vi "ClientTest.vi"() -> ()   [LabVIEW 2019]
panel:
  in  "port":u16
  in  "remote IP":string
  out "RawData":string
  in  "End":string="</CurrentMeasure>"
  out "CurrentData":string
  in  "Start":string="<CurrentMeasure>"
  out "error out TCPIP":errorcluster
  out "TM State Machine":string
  out "TM State Machine update time":timestamp
  out "TMisConnected":bool
  out "stopped":bool
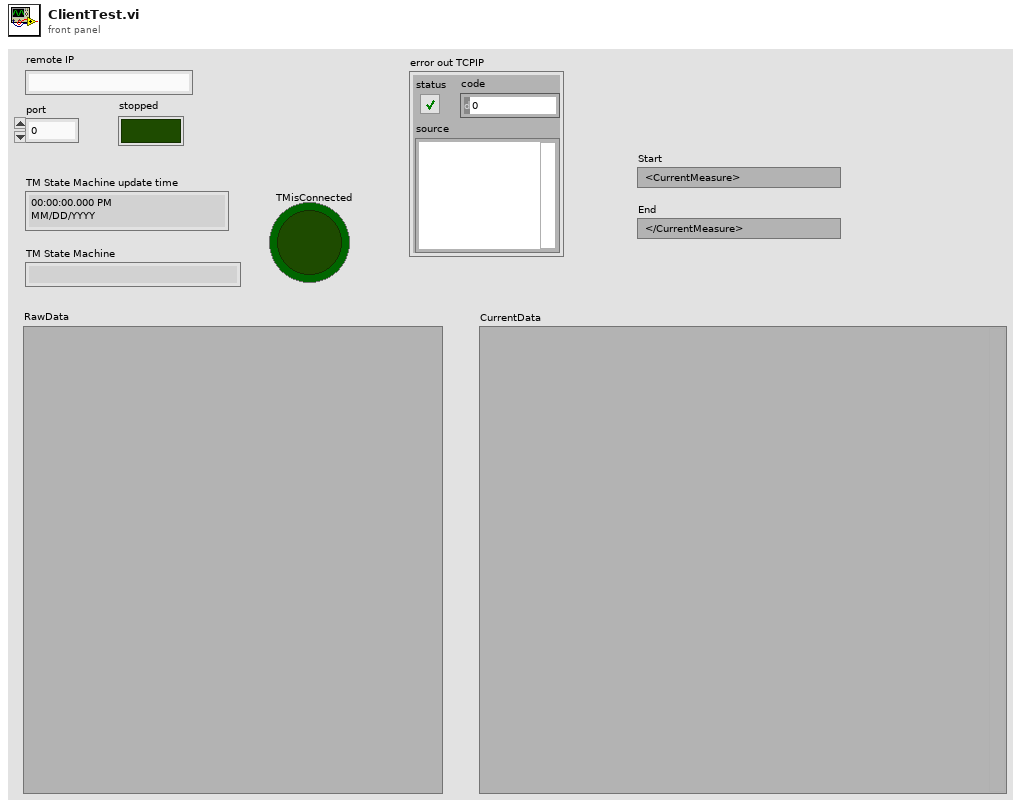
[diagram p1: front panel]
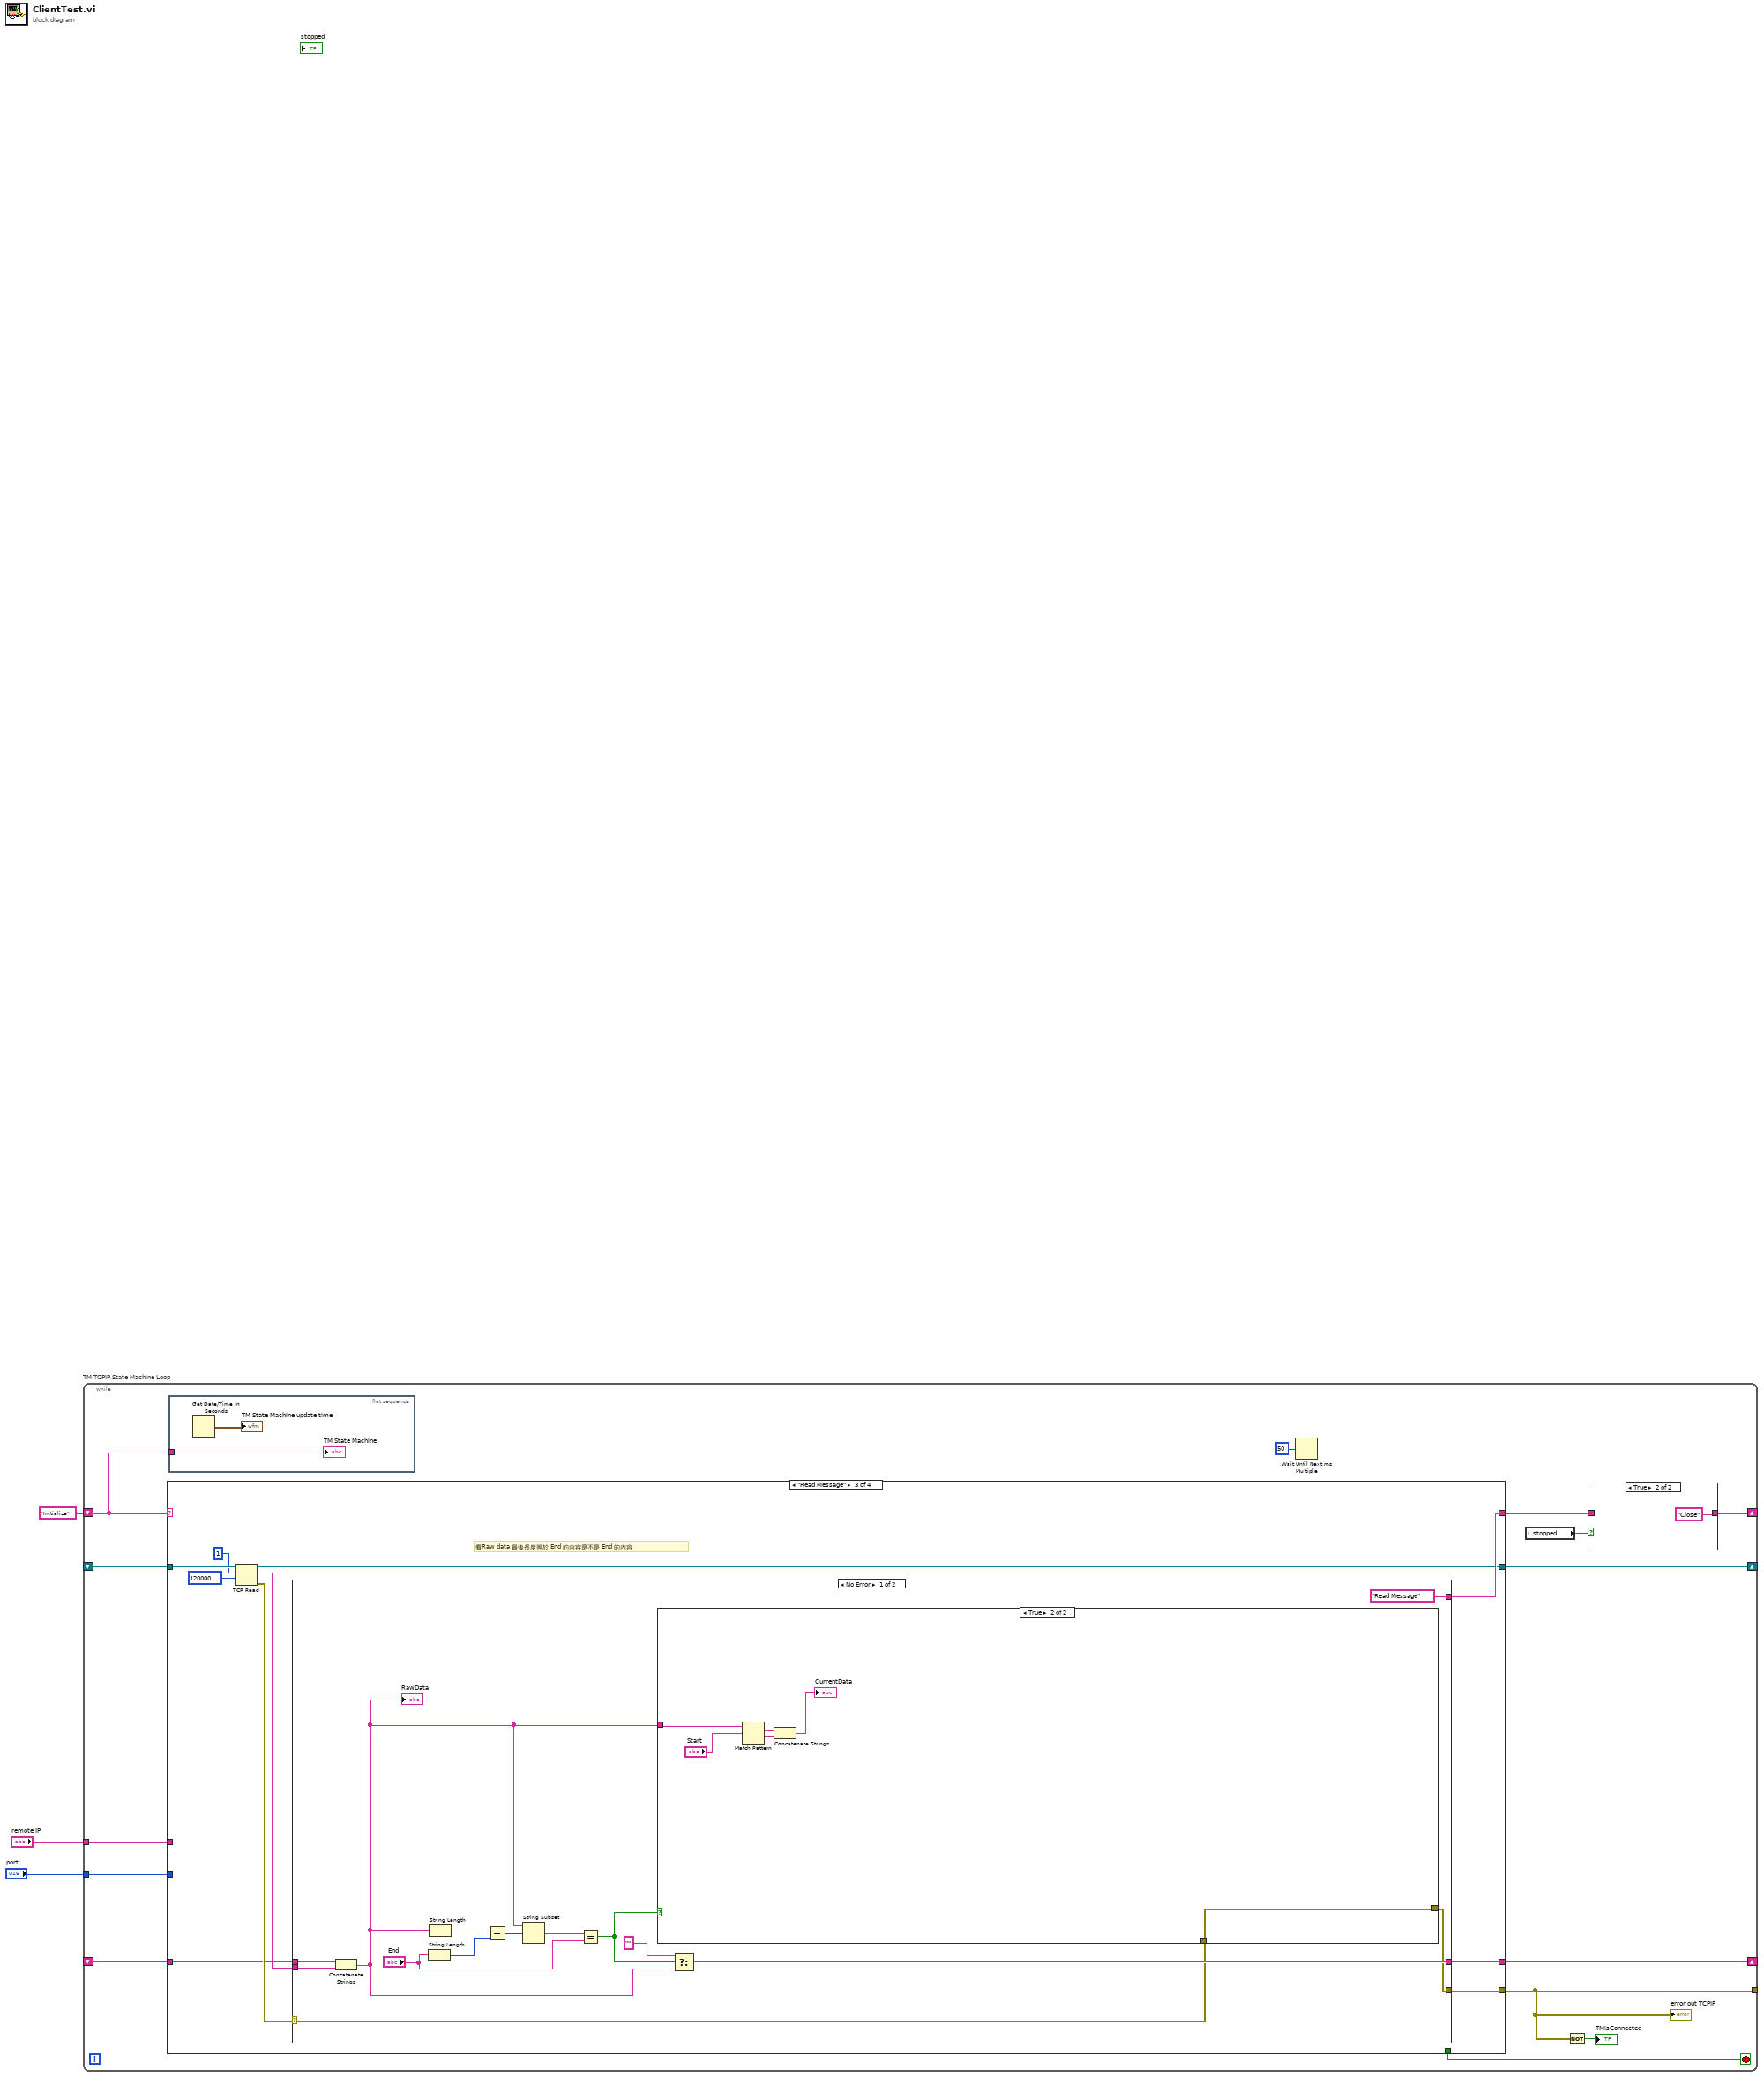
[diagram p0: block diagram]
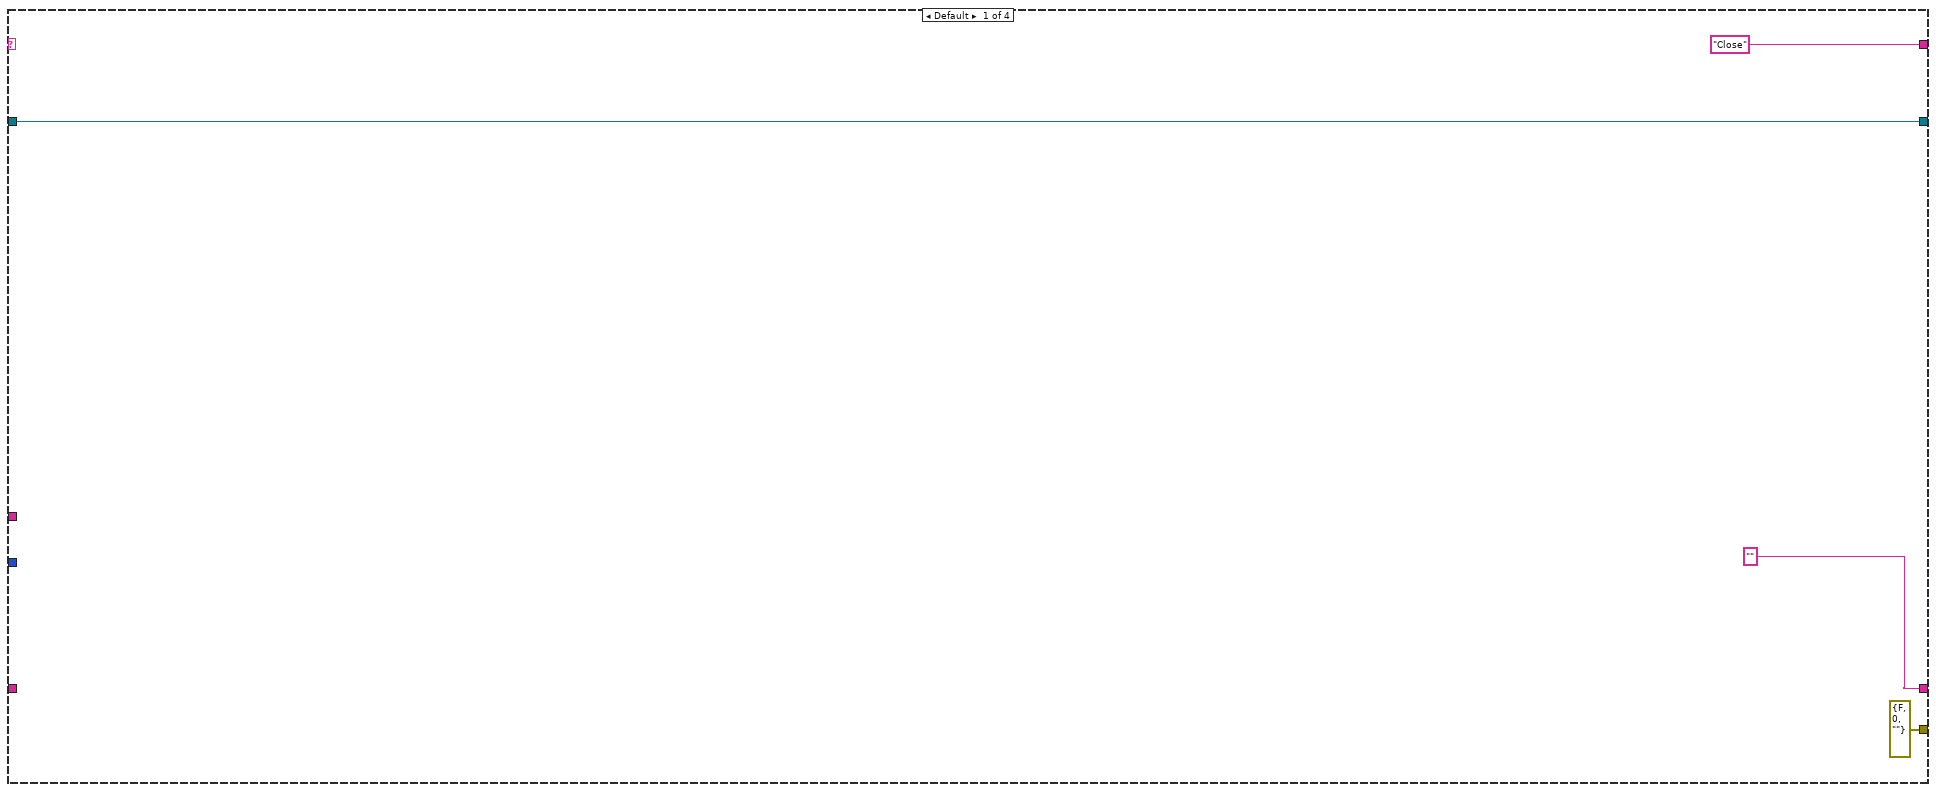
[diagram p3: hidden frame]
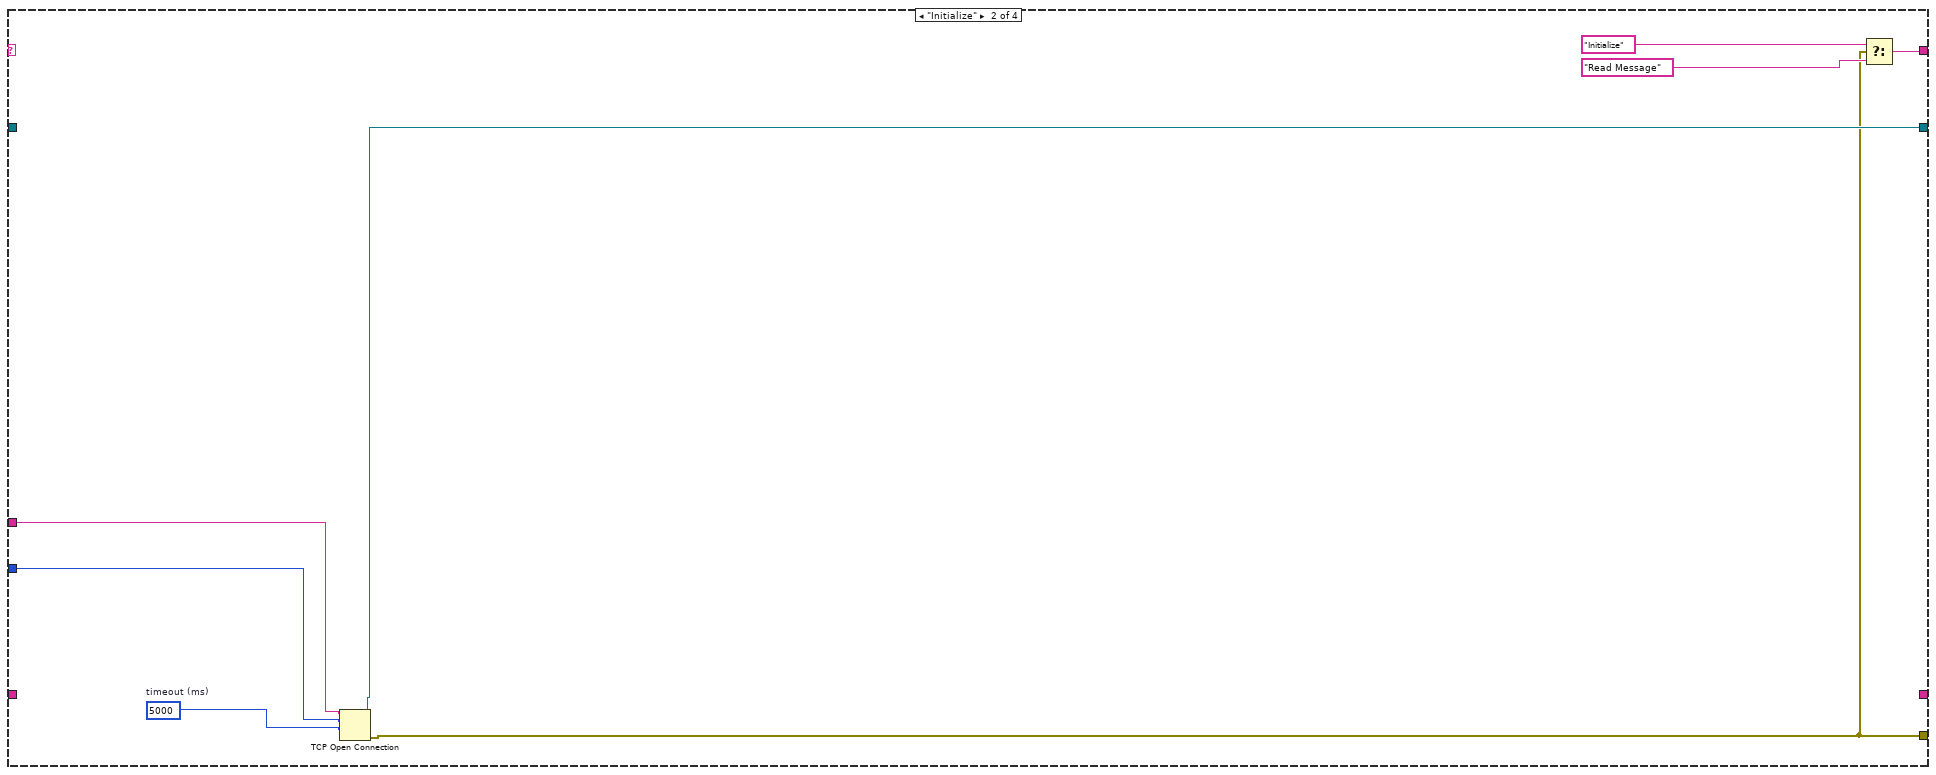
[diagram p4: hidden frame]
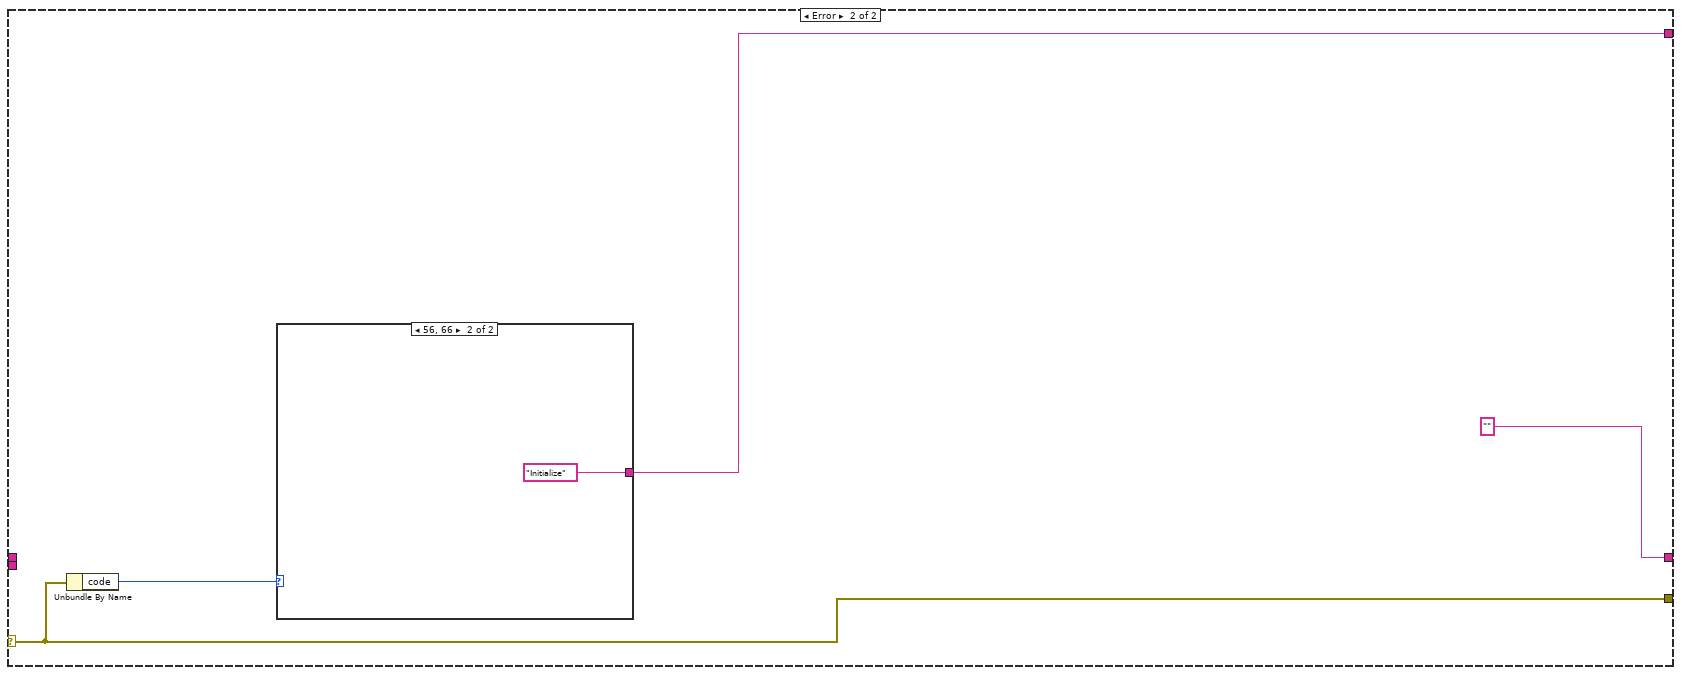
[diagram p6: hidden frame]
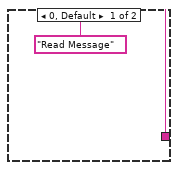
[diagram p7: hidden frame]
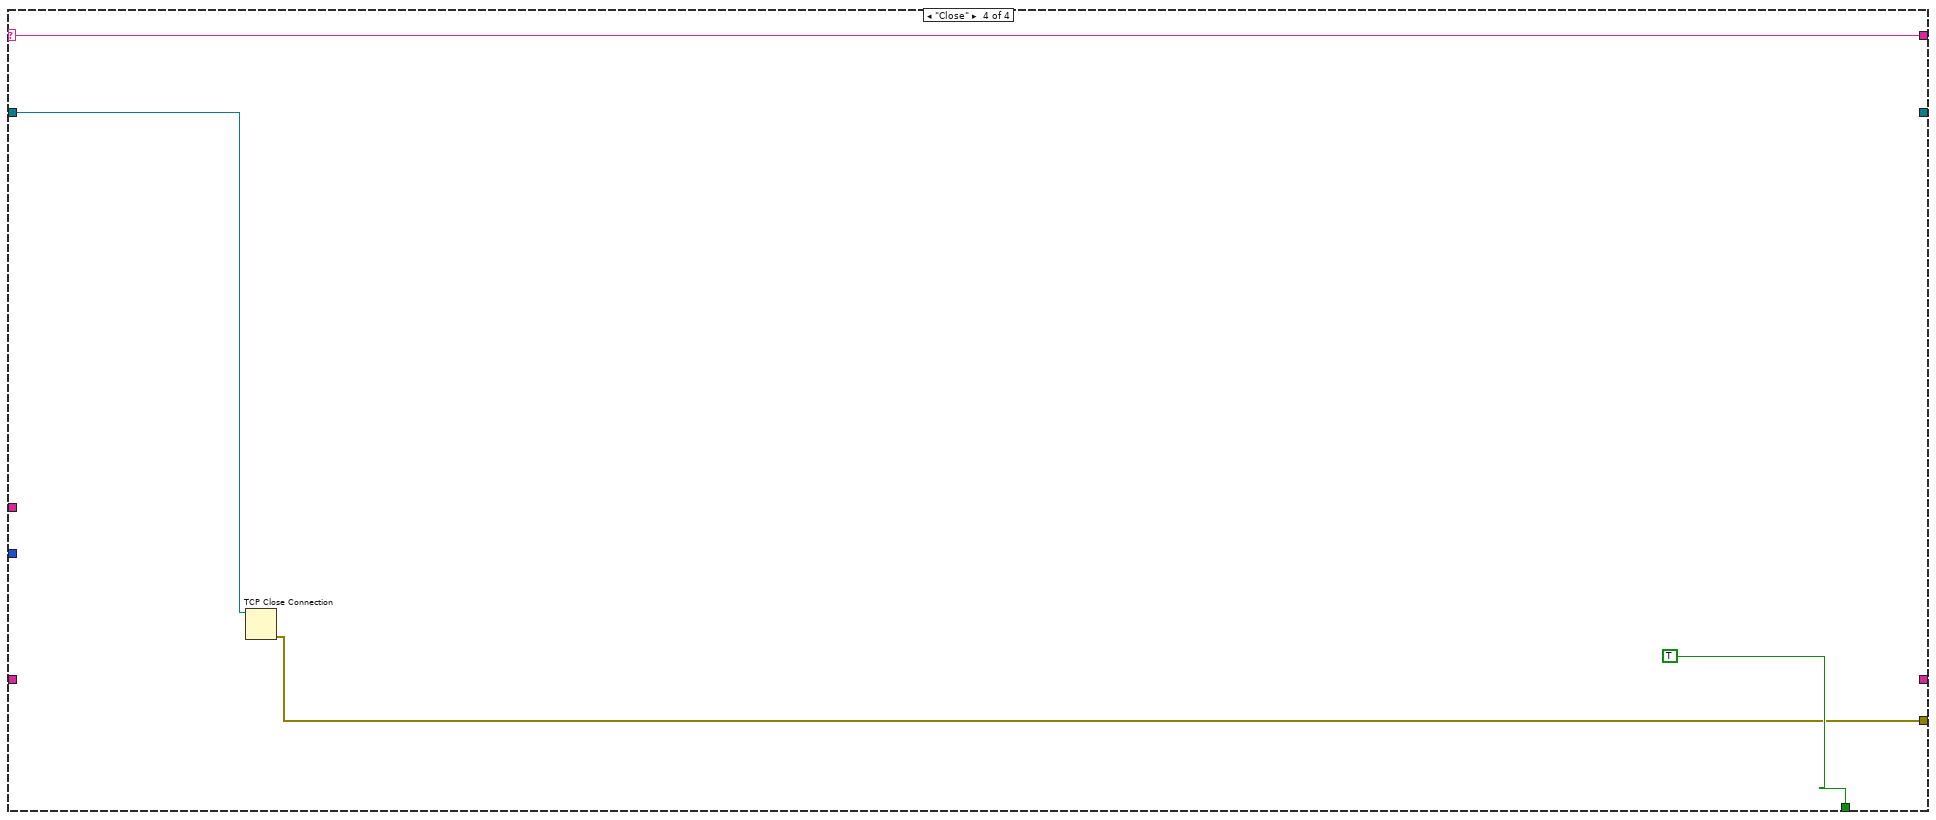
[diagram p8: hidden frame]
diagram:
  n1 = while "TM TCPIP State Machine Loop" {
    shift-right: [w10] -> _
    shift-left: "Initialize" -> [w9]
    tunnel: [w8] -> _
    shift-right: [w17] -> _
    shift-left: _ -> [w16]
    shift-right: [w15] -> _
    shift-left: _ -> [w14]
    tunnel: "remote IP" -> [w7]
    tunnel: "port" -> [w6]
    stop <- w13 stop-if-true
    n2 = case shown="\"Read Message\"" w9 {
      selector: w9 -> [_ _ _ w72]
      tunnel: ["Close" w31 w39 w72] -> w11
      tunnel: [errorcluster {"status"=FALSE, "code"=0, "source"=""} ("error out") w26 w34 w71] -> w8
      tunnel: [w25 w27 w38 _] -> w17
      tunnel: w16 -> [w25 _ w43 w74]
      tunnel: ["" _ w36 _] -> w15
      tunnel: w14 -> [_ _ w35 _]
      tunnel: [_ _ _ TRUE] -> w13
      tunnel: w7 -> [_ w30 _ _]
      tunnel: w6 -> [_ w29 _ _]
      frame Default {
      }
      frame "Initialize" {
        w28 = 5000  # timeout (ms)
        n3 = TCP Open Connection(address=w30, remote port or service name=w29, timeout ms (60000)=w28) -> (connection ID=w27:refnum<k5>, error out=w26:errorcluster)  [unwired: 2 in]
        n4 = Select(t="Initialize", s=w26, f="Read Message") -> (s? t:f=w31:string)
      }
      frame "Read Message" {
        # "看Raw data 最後長度等於 End 的內容是不是 End 的內容"
        n5 = TCP Read(connection ID=w43, bytes to read=1, 9:120000 ("timeout ms (25000)")) -> (connection ID out=w38:refnum<k5>, data out=w37:string, error out=w40:errorcluster)  [unwired: 2 in]
        n6 = case shown="No Error" w40 {
          selector: w40 -> [w46 w67]
          tunnel: ["Read Message" w65] -> w39
          tunnel: [w45 w67] -> w34
          tunnel: w37 -> [w51 _]
          tunnel: [w56 ""] -> w36
          tunnel: w35 -> [w52 _]
          frame No Error {
            n7 = Concatenate Strings(w52, w51) -> (w53:string)
            "RawData" <- w53
            n8 = String Length(string="End") -> (length=w50:i32)
            n9 = String Length(string=w53) -> (length=w55:i32)
            n10 = Subtract(x=w55, y=w50) -> (x-y=w48:i32)
            n11 = String Subset(string=w53, offset (0)=w48) -> (substring=w47:string)  [unwired: 1 in]
            n12 = Equal?(x=w47, y="End") -> (x = y?=w54:bool)
            n13 = case shown="True" w54 {
              tunnel: w53 -> [_ w63]
              tunnel: w46 -> [w58 w59]
              tunnel: [w58 w59] -> w45
              frame False {
              }
              frame True {
                n14 = Match Pattern(string=w63, regular expression="Start") -> (match substring=w62:string, after substring=w61:string)  [unwired: 1 in, 2 out]
                n15 = Concatenate Strings(w62, w61) -> (→"CurrentData":string)
              }
            }
            n16 = Select(t="", s=w54, f=w53) -> (s? t:f=w56:string)
          }
          frame Error {
            n17 = Unbundle By Name(w67) -> ("code"=w66:i32)
            n18 = case shown="56, 66" w66 {
              tunnel: ["Read Message" "Initialize"] -> w65
              frame 0, Default {
              }
              frame 56, 66 {
              }
            }
          }
        }
      }
      frame "Close" {
        n19 = TCP Close Connection(connection ID=w74) -> (error out=w71:errorcluster)  [unwired: 1 in, 2 out]
      }
    }
    "error out TCPIP" <- w8
    n20 = flat-sequence {
      tunnel: w9 -> [w19]
      frame #0 {
        n21 = Get Date/Time In Seconds() -> (seconds since 1Jan1904=→"TM State Machine update time":timestamp)
        "TM State Machine" <- w19
      }
    }
    n22 = Wait Until Next ms Multiple(millisecond multiple=u32 50) -> ()  [unwired: 1 out]
    n23 = local read "stopped"() -> (w12:bool)
    n24 = Not(x=w8) -> (.not. x?=→"TMisConnected":bool)
    n25 = case shown="True" w12 {
      tunnel: w11 -> [w20 _]
      tunnel: [w20 "Close"] -> w10
      frame False {
      }
      frame True {
      }
    }
  }
